vi "from_reference.vi"(8 "error in (no error)":errorcluster, 10 "ref":u64) -> (0 "error out":errorcluster, 3 "Table out":refnum<class "Table.lvclass">)   [LabVIEW 2020, in "toml_edit.lvlib" / "Table.lvclass"]
uses:
  Table.lvclass
  Table.lvclass/Table.ctl
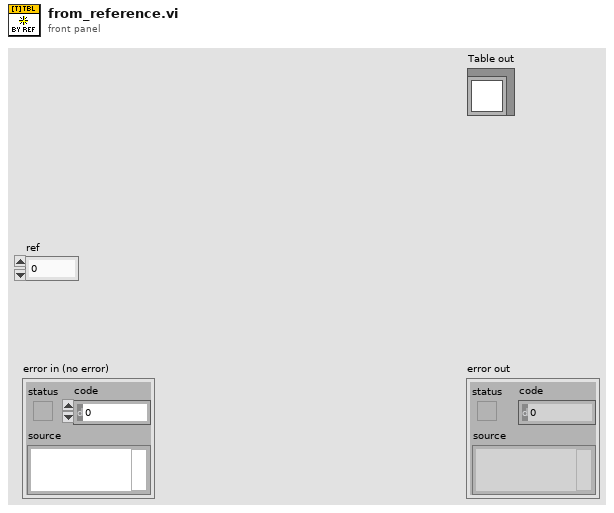
[diagram p1: front panel]
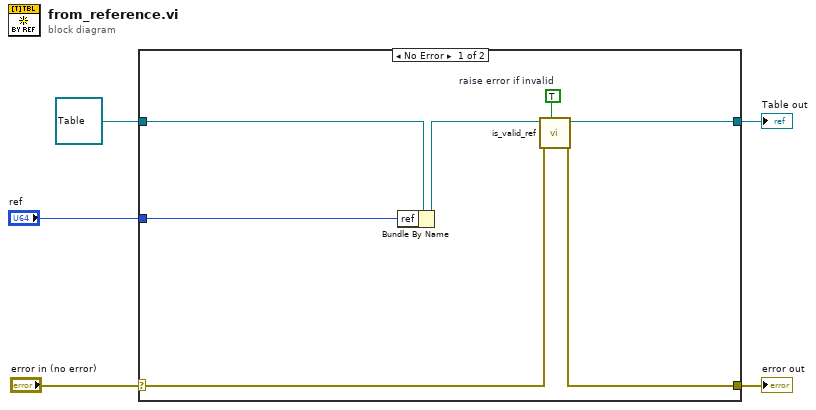
[diagram p0: block diagram]
diagram:
  n1 = case shown="No Error" "error in (no error)" {
    selector: "error in (no error)" -> [w7 w14]
    tunnel: [w6 w14] -> w4
    tunnel: [w8 w13] -> w2
    tunnel: refnum<class "Table.lvclass"> refnum ("Table in") -> [w12 w13]
    tunnel: "ref" -> [w11 _]
    frame No Error {
      w10 = TRUE  # raise error if invalid
      n2 = Bundle By Name(cluster=w12, "ref"=w11) -> (w9:refnum<class "Table.lvclass">)
      n3 = call-dynamic "is_valid_ref.vi"("raise error if invalid? (False)"=w10, "error in (no error)"=w7, "Table in"=w9) -> ("error out"=w6:errorcluster, "Table out"=w8:refnum<class "Table.lvclass">)  [unwired: 6 in, 1 out]
    }
    frame Error {
    }
  }
  "error out" <- w4
  "Table out" <- w2
